vi "MSScript_Format_UpdConj.vi"(9 "ValueArray":string[](array[string]), 10 "TagArray":string[](array[string]), 11 "MSScript.lvclass":refnum<class "MSScript.lvclass">) -> (0 "ValueErrorArray":bool[](array[boolean]), 1 "TagErrorArray":bool[](array[boolean]), 2 "ParamErrorArray":bool[](array[boolean]), 3 "Data":variant, 4 "#ofParamError":bool)   [LabVIEW 2018, in "MSScript.lvclass"]
uses:
  MSScript.lvclass
  Ctl/MSEditorParam updConj.ctl
  MSScript_Transform_UInt.vi
  MSScript_Transform_Boolean.vi
  MSScript_Transform_UIntArray.vi
  MSScript_Transform_EXTArray.vi
panel:
  in  "ParamValueType":T1={"iniPhase"=2147483648, "conjLen"=[3.0, 3.0], "phaseDiff"=[2147483648, 2147483648], "fixedLen"=FALSE}
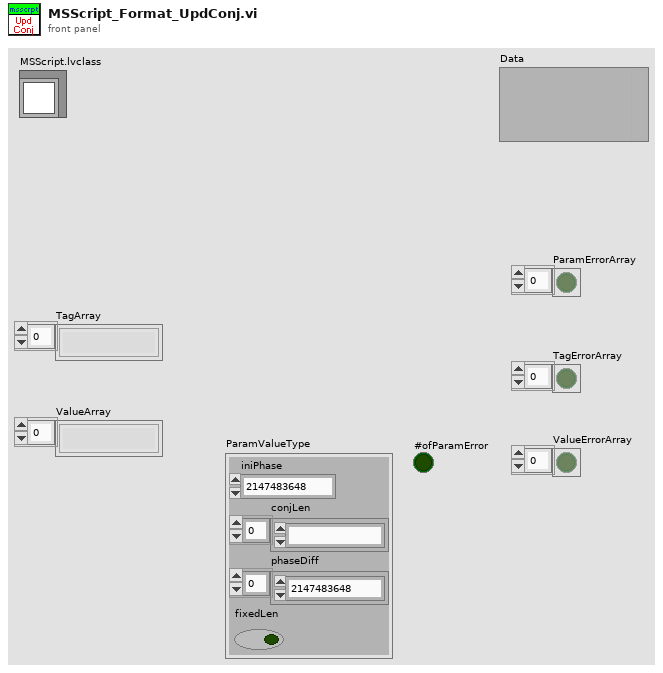
[diagram p1: front panel]
types:
  T1 = typedef "MSEditorParam updConj.ctl" = cluster{"iniPhase":u32, "conjLen":ext[], "phaseDiff":u64[], "fixedLen":bool}
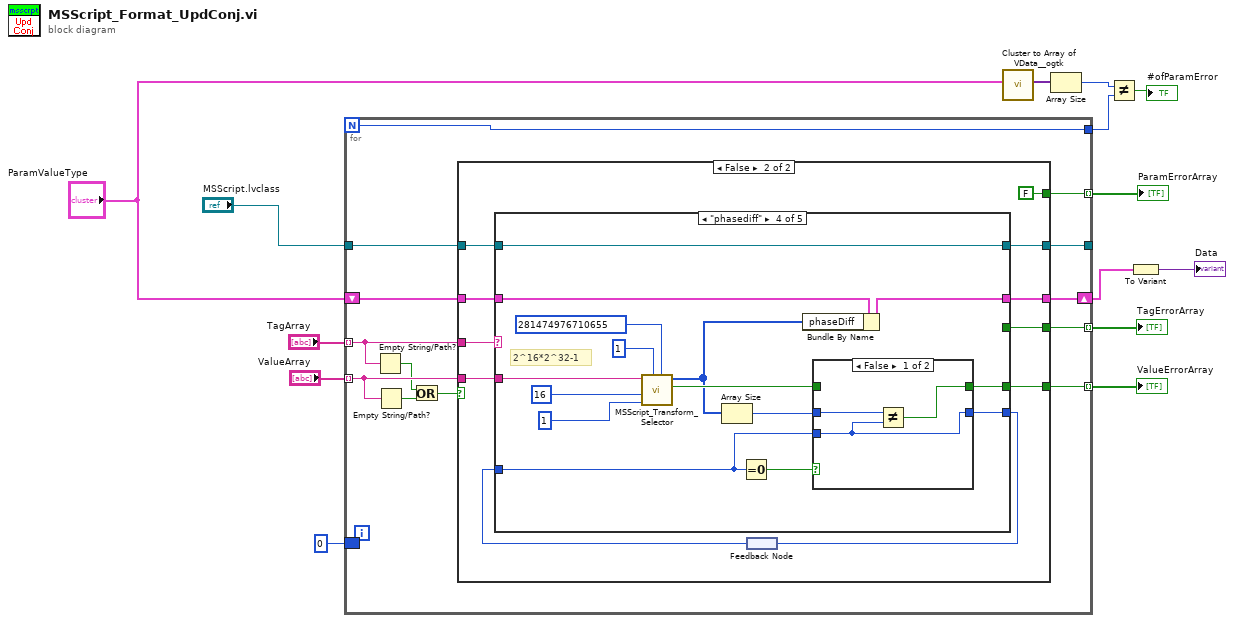
[diagram p0: block diagram]
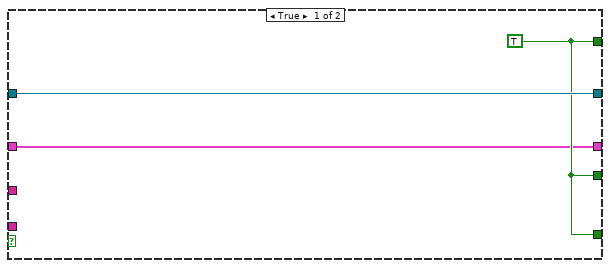
[diagram p2: hidden frame]
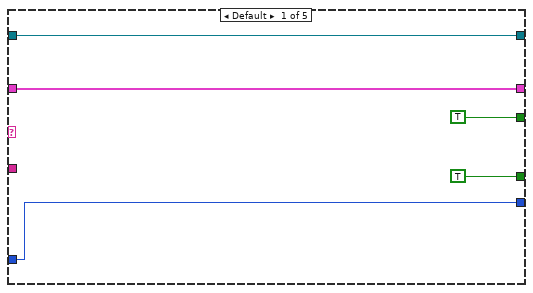
[diagram p3: hidden frame]
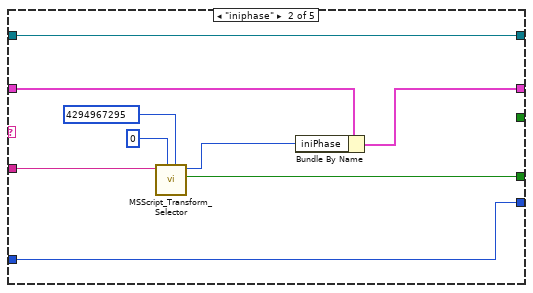
[diagram p4: hidden frame]
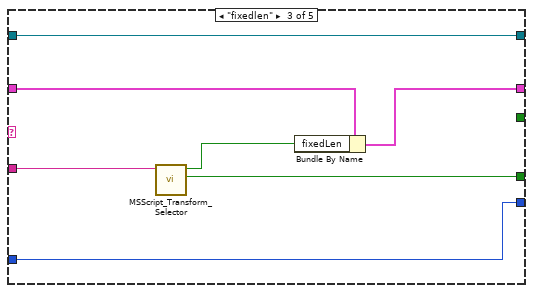
[diagram p5: hidden frame]
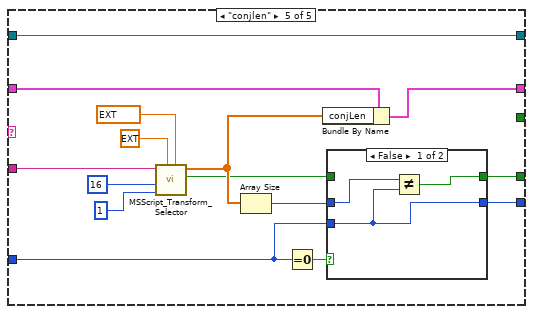
[diagram p7: hidden frame]
diagram:
  n1 = for {
    N -> [w15]
    tunnel: "TagArray" -> [w24] mode=indexing
    tunnel: "ValueArray" -> [w23] mode=indexing
    tunnel: [w16] -> w12 mode=indexing
    tunnel: "MSScript.lvclass" -> [w27]
    tunnel: [w26] -> w13 mode=indexing
    tunnel: [w25] -> _
    tunnel: [w19] -> w14 mode=indexing
    shift-right: [w17] -> w2
    shift-left: "ParamValueType" -> [w18]
    tunnel: [w15] -> w4
    border: 0 -> [_]
    n2 = Empty String/Path?(string/path=w24) -> (empty?=w21:bool)
    n3 = Empty String/Path?(string/path=w23) -> (empty?=w22:bool)
    n4 = Or(x=w21, y=w22) -> (x .or. y?=w20:bool)
    n5 = case shown="False" w20 {
      tunnel: w27 -> [w30 w40]
      tunnel: [w29 w36] -> w26
      tunnel: [w30 w33] -> w25
      tunnel: w24 -> [_ w38]
      tunnel: w23 -> [_ w37]
      tunnel: [w29 FALSE] -> w19
      tunnel: w18 -> [w28 w39]
      tunnel: [w28 w34] -> w17
      tunnel: [w29 w35] -> w16
      frame True {
        w29 = TRUE
      }
      frame False {
        n6 = feedback #1() -> (w32:i32)
        n7 = case shown="\"phasediff\"" w38 {
          tunnel: [TRUE _ _ _ _] -> w35
          tunnel: w40 -> [w44 w53 w60 w76 w96]
          tunnel: w37 -> [_ w54 w61 w77 w97]
          tunnel: [TRUE ("Value Error?") w55 w62 w69 w87] -> w36
          tunnel: [w44 w53 w60 w76 w96] -> w33
          tunnel: w39 -> [w43 w51 w58 w75 w95]
          tunnel: [w43 w50 w57 w74 w94] -> w34
          tunnel: [w42 w47 w56 w64 w84] -> w31
          tunnel: w32 -> [w42 w47 w56 w63 w83]
          frame Default {
          }
          frame "iniphase" {
            n8 = call-poly "MSScript_Transform_Selector.vi"("upper limit"=u64 4294967295, "lower limit"=u64 0, "string in"=w54) -> ("Value Error?"=w55:bool, "Value Output"=w52:u64)  [unwired: 6 in, 1 out]
            n9 = Bundle By Name(cluster=w51, "iniPhase"=w52) -> (w50:T1)
          }
          frame "fixedlen" {
            n10 = call-poly "MSScript_Transform_Selector.vi"("Check_Str"=w61) -> ("Value Error?"=w62:bool, "Value Output"=w59:bool)  [unwired: 9 in]
            n11 = Bundle By Name(cluster=w58, "fixedLen"=w59) -> (w57:T1)
          }
          frame "phasediff" {
            # "2^16*2^32-1"
            n12 = call-poly "MSScript_Transform_Selector.vi"("upper limit (18446744073709551615)"=u64 281474976710655 ("upper limit"), "lower limit (0)"=u64 1 ("lower limit"), "MinSize"=1, "MaxSize"=16, "Check_Str"=w77) -> ("Value Error?"=w68:bool, "Value Output"=w65:u64[])  [unwired: 4 in, 1 out]
            n13 = Array Size(array=w65) -> (size(s)=w66:i32)
            n14 = Equal To 0?(x=w63) -> (x = 0?=w67:bool)
            n15 = Bundle By Name(cluster=w75, "phaseDiff"=w65) -> (w74:T1)
            n16 = case shown="False" w67 {
              tunnel: w66 -> [w80 w81]
              tunnel: [w79 w82] -> w69
              tunnel: w68 -> [_ w82]
              tunnel: [w78 w81] -> w64
              tunnel: w63 -> [w78 _]
              frame False {
                n17 = Not Equal?(x=w80, y=w78) -> (x != y?=w79:bool)
              }
              frame True {
              }
            }
          }
          frame "conjlen" {
            n18 = call-poly "MSScript_Transform_Selector.vi"("upper limit (Inf)"=ext 49.999 ("upper limit"), "lower limit (-Inf)"=ext 0.0 ("lower limit"), "MinSize"=u8 1, "MaxSize"=u8 16, "check_str"=w97) -> ("Value Error?"=w88:bool, "Value Output"=w89:ext[])  [unwired: 4 in, 1 out]
            n19 = Array Size(array=w89) -> (size(s)=w85:i32)
            n20 = Equal To 0?(x=w83) -> (x = 0?=w86:bool)
            n21 = Bundle By Name(cluster=w95, "conjLen"=w89) -> (w94:T1)
            n22 = case shown="False" w86 {
              tunnel: w85 -> [w100 w101]
              tunnel: [w99 w102] -> w87
              tunnel: w88 -> [_ w102]
              tunnel: [w98 w101] -> w84
              tunnel: w83 -> [w98 _]
              frame False {
                n23 = Not Equal?(x=w100, y=w98) -> (x != y?=w99:bool)
              }
              frame True {
              }
            }
          }
        }
        n24 = feedback-in #1(w31) -> ()
      }
    }
  }
  "TagErrorArray" <- w12
  "ValueErrorArray" <- w13
  "ParamErrorArray" <- w14
  n25 = call <userlib>:"Cluster to Array of VData__ogtk.vi"("Cluster"="ParamValueType") -> ("Array of VData"=w8:variant[])  [unwired: 9 in, 1 out]
  n26 = Array Size(array=w8) -> (size(s)=w7:i32)
  n27 = Not Equal?(x=w7, y=w4) -> (x != y?=→"#ofParamError":bool)
  n28 = To Variant(anything=w2) -> (Variant=→"Data":variant)
